vi "Wavenames and comments.vi"(11 "Path":path) -> (2 "Notes":string, 3 "Array":string[][](array[string]))   [LabVIEW 2016]
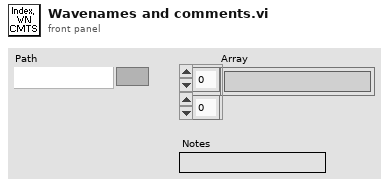
[diagram p1: front panel]
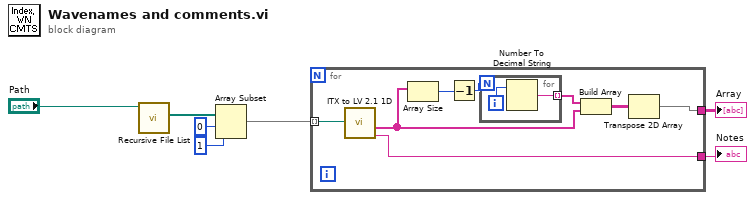
[diagram p0: block diagram]
diagram:
  n1 = call <vilib>:"Recursive File List.vi"("Folder Path"="Path") -> ("All Files in Dir"=w1:path[])  [unwired: 7 in, 3 out]
  n2 = Array Subset(array=w1, index=0, length=1) -> (w4:path[])
  n3 = for {
    tunnel: w4 -> [w11] mode=indexing
    tunnel: [w9] -> w6
    tunnel: [w8] -> w7
    n4 = call <userlib>:"ITX to LV 2.1 1D.vi"("file (use dialog)"=w11) -> ("wave names"=w10:string[], "Notes"=w8:string)  [unwired: 2 in, 1 out]
    n5 = Array Size(array=w10) -> (size(s)=w13:i32)
    n6 = Decrement(x=w13) -> (x-1=w14:i32)
    n7 = for {
      N: w14 -> [_]
      tunnel: [w16] -> w12 mode=indexing
      i -> [w17]
      n8 = Number To Decimal String(number=w17) -> (decimal integer string=w16:string)  [unwired: 1 in]
    }
    n9 = Build Array(w12, w10) -> (w15:string[][])
    n10 = Transpose 2D Array(2D array=w15) -> (transposed array=w9:string[][])
  }
  "Notes" <- w7
  "Array" <- w6
